vi "Sample 34401A Measurement.vi"(0 "VISA resource name":refnum<visa-resource-name>, 5 "Function (0: DC Voltage)":u16(ring) items=["DC Voltage", "AC Voltage", "2 - Wire Resistance", "4 - Wire Resistance", "DC Current", "AC Current", "Frequency", "Period", "Continuity", "Diode Checking", "VDC:VDC Ratio", "Temperature", "Capacitance"], 7 "Wire Mode (1: 4-Wire)":i16(ring)=1 items=["2-Wire", "4-Wire"], 9 "Unit (0: Celsius)":u16(ring) items=["C", "F", "K"], 11 "error in":errorcluster) -> (4 "Measurement":dbl, 15 "error out":errorcluster)   [LabVIEW 2021]
uses:
  <instrlib>/Agilent 34401/Public/Configure/Configure Temperature (RTD).vi
  <instrlib>/Agilent 34401/Public/Data/Read (Single Point).vi
  <instrlib>/Agilent 34401/Agilent 34401.lvlib
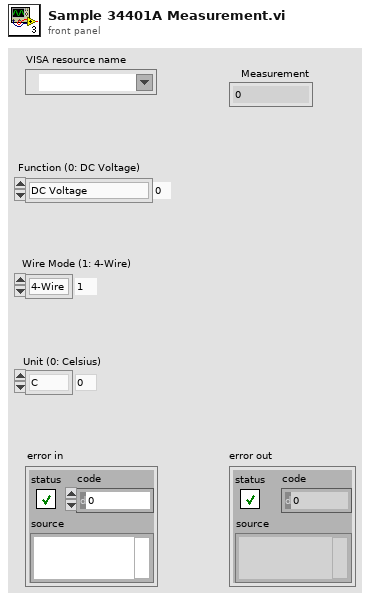
[diagram p1: front panel]
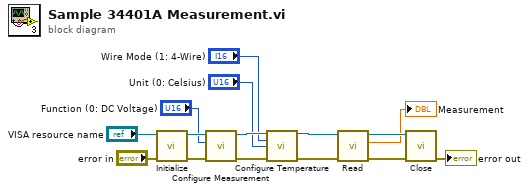
[diagram p0: block diagram]
diagram:
  n1 = call <instrlib>:"Initialize.vi"("error in (no error)"="error in", "VISA resource name"="VISA resource name") -> ("error out"=w11:errorcluster, "VISA resource name out"=w15:refnum<visa-resource-name>)  [unwired: 8 in]
  n2 = call <instrlib>:"Configure Measurement.vi"("error in (no error)"=w11, "Function (0: DC Voltage)"="Function (0: DC Voltage)", "VISA resource name"=w15) -> ("error out"=w10:errorcluster, "VISA resource name out"=w14:refnum<visa-resource-name>)  [unwired: 7 in]
  n3 = call-poly <instrlib>:"Configure Temperature.vi"("VISA resource name"=w14, "Wire Mode (1: 4-Wire)"="Wire Mode (1: 4-Wire)", "Unit (0: Celsius)"="Unit (0: Celsius)", "error in (no error)"=w10) -> ("VISA resource name out"=w13:refnum<visa-resource-name>, "error out"=w9:errorcluster)  [unwired: 10 in]
  n4 = call-poly <instrlib>:"Read.vi"("error in (no error)"=w9, "VISA resource name"=w13) -> ("error out"=w8:errorcluster, "Measurement"=→"Measurement":dbl, "VISA resource name out"=w12:refnum<visa-resource-name>)  [unwired: 7 in]
  n5 = call <instrlib>:"Close.vi"("error in (no error)"=w8, "VISA resource name"=w12) -> ("error out"=→"error out":errorcluster)  [unwired: 9 in]
